vi "Read_Write_Beam_Data.vi"(1 "Beam Data In":T2={"Vg1 (Green 1 dir. vect.)"=[0.059117350659853476, -0.996541267827751, 0.05840068807144843], "Vg2  (Green 2 dir. vect.)"=[-0.05232536310393669, -0.9971561380468801, -0.054237373935992664], "Vb1 (Blue 1 dir. vect.)"=[-0.052923229613528855, -0.9969242065933935, 0.057803616456121795], "Vb2 (Blue 1 dir. vect.)"=[0.05971521716944564, -0.9967731992812374, -0.05364030232066602], "Porb (Orb XYZ posn. forced coplanar)"=[2201.0738225655555, -1199.3737231995547, 269.758310600838], "Porb (Orb XYZ posn. - allow skew)"=[2200.796256301178, -1199.3740953152687, 270.0329332816893], "Orb posn. uncertainty, +/- dx, dy, dz"=[0.13878313218879157, 0.00018605785703584843, 0.13731134042564008], "Vp (Actual Probe dir. vect)"=[0.003406702197773746, -0.9999920168246164, 0.0020882210543692924], "Yaw (deg)"=89.80480953887573, "Pitch (deg)"=0.11964634006213794, "In-Plane Roll (deg)"=45.305328966424156, "Beam Half Angle (deg)"=4.544091484248422, "B1 Close P11"=[0.0, 0.0, 0.0], "B1 Far P12"=[2158.01, -491.04, 229.28], "B2 Close P22"=[2158.01, -491.04, 229.28], "B2 Far P21"=[2158.01, -491.04, 229.28], "Projected Roll (deg)"=0.0, "Green Velocity Vector"=[0.0, 0.0, 0.0], "Blue Velocity Vector"=[0.0, 0.0, 0.0], "Probe is facing...."="-", "Calculation Method"=""} {"Vp (Actual Probe dir. vect)" format="%#_6f"; "Vg2  (Green 2 dir. vect.)" format="%#_6f"; "Vg1 (Green 1 dir. vect.)" format="%#_6f"}, 2 "Mode":T1(ring)) -> (0 "Beam Data Out":T2={"Vg1 (Green 1 dir. vect.)"=[0.059117350659853476, -0.996541267827751, 0.05840068807144843], "Vg2  (Green 2 dir. vect.)"=[-0.05232536310393669, -0.9971561380468801, -0.054237373935992664], "Vb1 (Blue 1 dir. vect.)"=[-0.052923229613528855, -0.9969242065933935, 0.057803616456121795], "Vb2 (Blue 1 dir. vect.)"=[0.05971521716944564, -0.9967731992812374, -0.05364030232066602], "Porb (Orb XYZ posn. forced coplanar)"=[2201.0738225655555, -1199.3737231995547, 269.758310600838], "Porb (Orb XYZ posn. - allow skew)"=[2200.796256301178, -1199.3740953152687, 270.0329332816893], "Orb posn. uncertainty, +/- dx, dy, dz"=[0.13878313218879157, 0.00018605785703584843, 0.13731134042564008], "Vp (Actual Probe dir. vect)"=[0.003406702197773746, -0.9999920168246164, 0.0020882210543692924], "Yaw (deg)"=89.80480953887573, "Pitch (deg)"=0.11964634006213794, "In-Plane Roll (deg)"=45.305328966424156, "Beam Half Angle (deg)"=4.544091484248422, "B1 Close P11"=[0.0, 0.0, 0.0], "B1 Far P12"=[2158.01, -491.04, 229.28], "B2 Close P22"=[2158.01, -491.04, 229.28], "B2 Far P21"=[2158.01, -491.04, 229.28], "Projected Roll (deg)"=0.0, "Green Velocity Vector"=[0.0, 0.0, 0.0], "Blue Velocity Vector"=[0.0, 0.0, 0.0], "Probe is facing...."="-", "Calculation Method"=""} {"Vp (Actual Probe dir. vect)" format="%#_6f"; "Vg2  (Green 2 dir. vect.)" format="%#_6f"; "Vg1 (Green 1 dir. vect.)" format="%#_6f"})   [LabVIEW 2010]
uses:
  Controls/LDA_Beam_Cluster.ctl
  File/Setup_Filetype.ctl
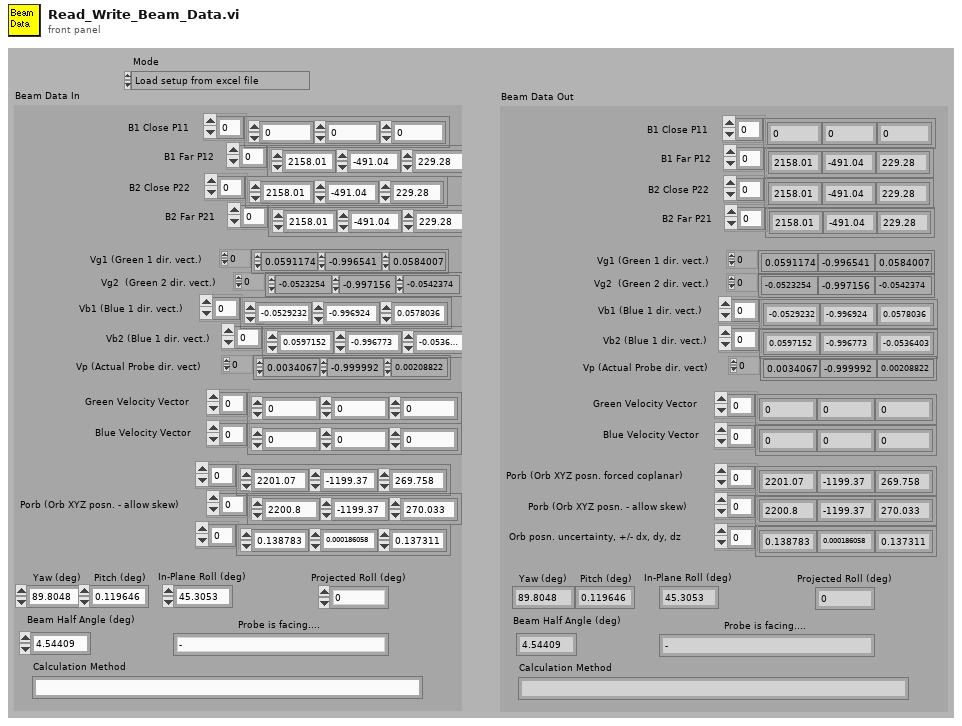
[diagram p1: front panel]
types:
  T1 = enum16{"Load setup from excel file", "Save setup to excel file"}
  T2 = typedef "LDA_Beam_Cluster.ctl" = cluster{"Vg1 (Green 1 dir. vect.)":dbl[], "Vg2  (Green 2 dir. vect.)":dbl[], "Vb1 (Blue 1 dir. vect.)":dbl[], "Vb2 (Blue 1 dir. vect.)":dbl[], "Porb (Orb XYZ posn. forced coplanar)":dbl[], "Porb (Orb XYZ posn. - allow skew)":dbl[], "Orb posn. uncertainty, +/- dx, dy, dz":dbl[], "Vp (Actual Probe dir. vect)":dbl[], "Yaw (deg)":dbl, "Pitch (deg)":dbl, "In-Plane Roll (deg)":dbl, "Beam Half Angle (deg)":dbl, "B1 Close P11":dbl[], "B1 Far P12":dbl[], "B2 Close P22":dbl[], "B2 Far P21":dbl[], "Projected Roll (deg)":dbl, "Green Velocity Vector":dbl[], "Blue Velocity Vector":dbl[], "Probe is facing....":string, "Calculation Method":string}
  T3 = typedef "Setup_Filetype.ctl" = enum16{"Measurement Setups", "Calibration Setups", "General", "Results File Plotter Setups", "Speed Calib Tweaks"}
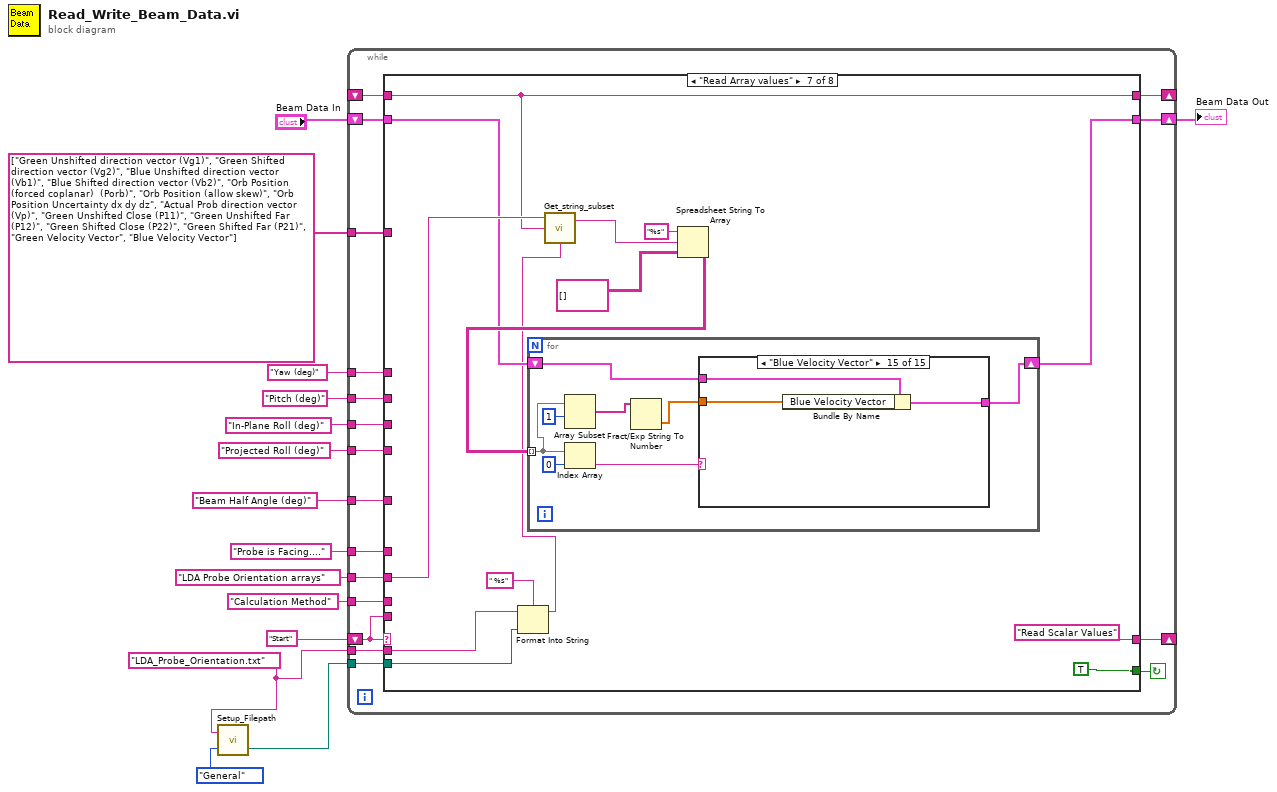
[diagram p0: block diagram]
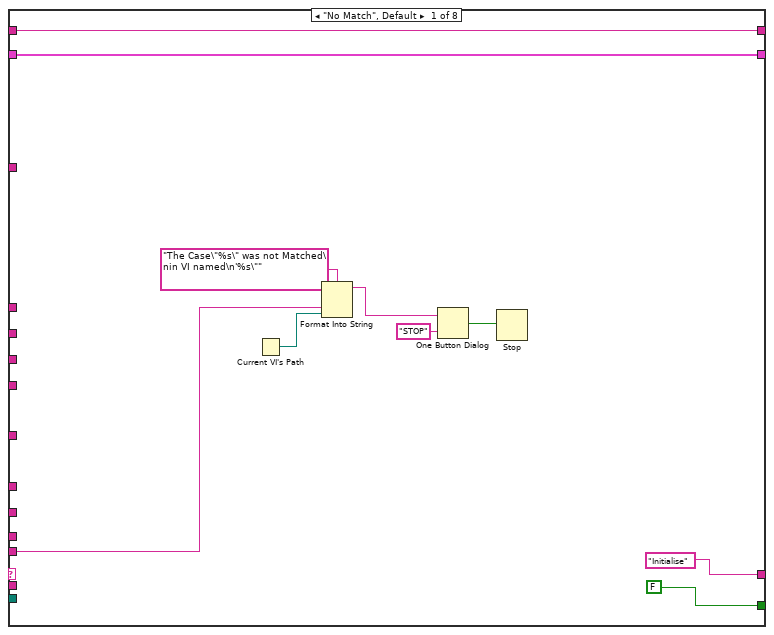
[diagram p2: hidden frame]
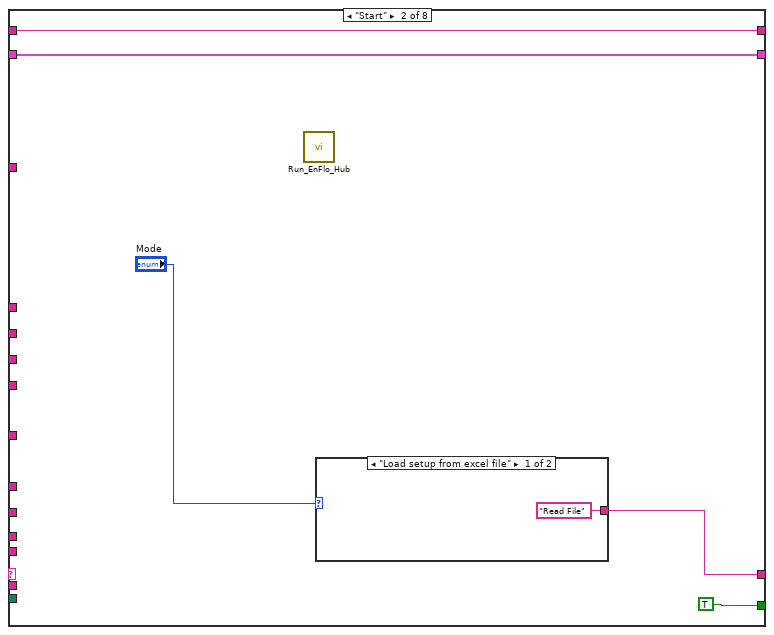
[diagram p3: hidden frame]
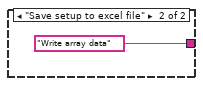
[diagram p4: hidden frame]
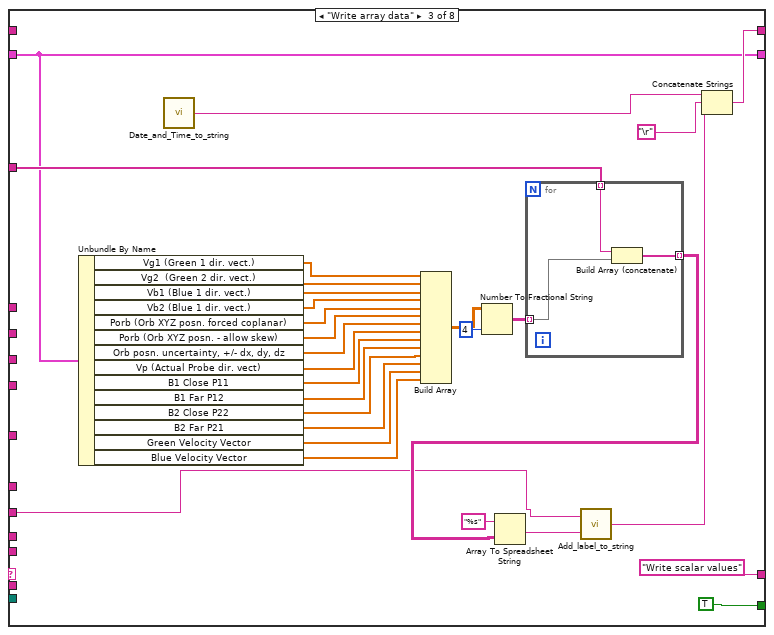
[diagram p5: hidden frame]
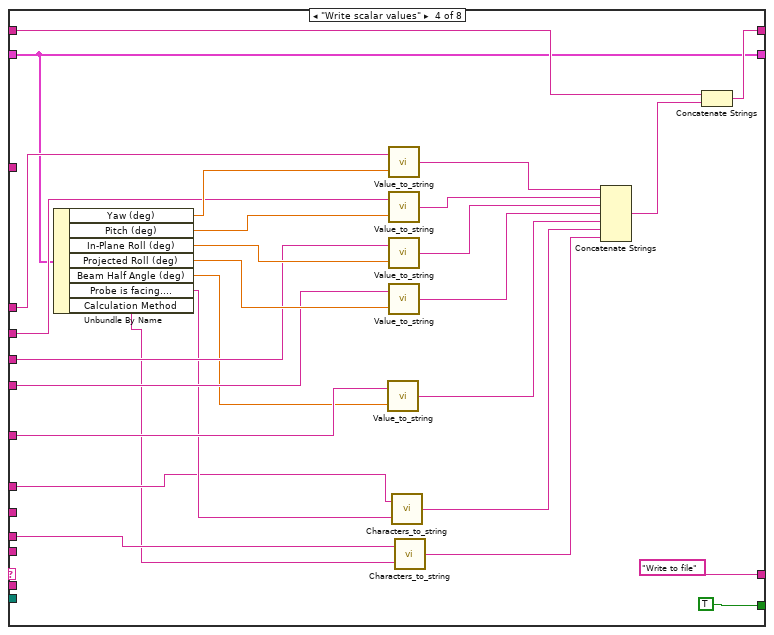
[diagram p6: hidden frame]
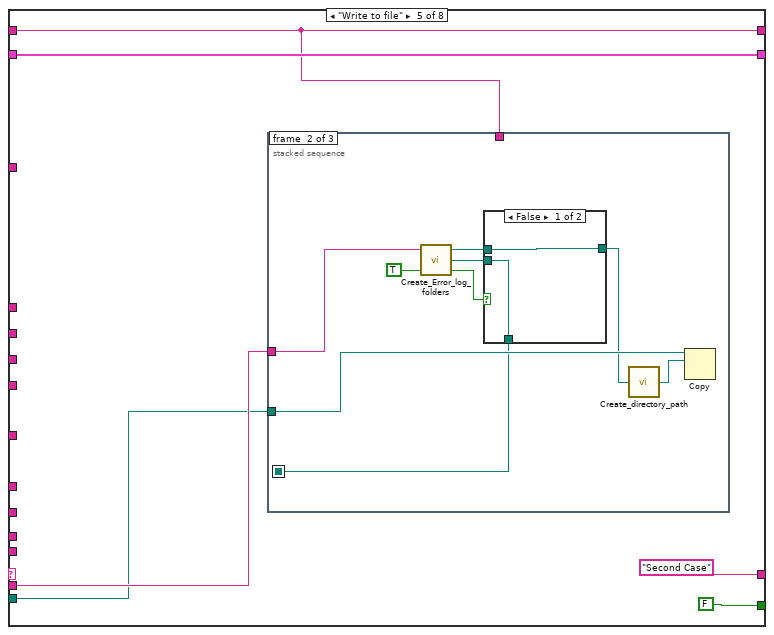
[diagram p7: hidden frame]
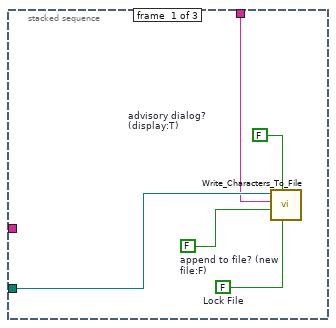
[diagram p8: hidden frame]
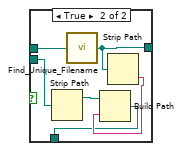
[diagram p9: hidden frame]
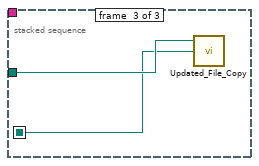
[diagram p10: hidden frame]
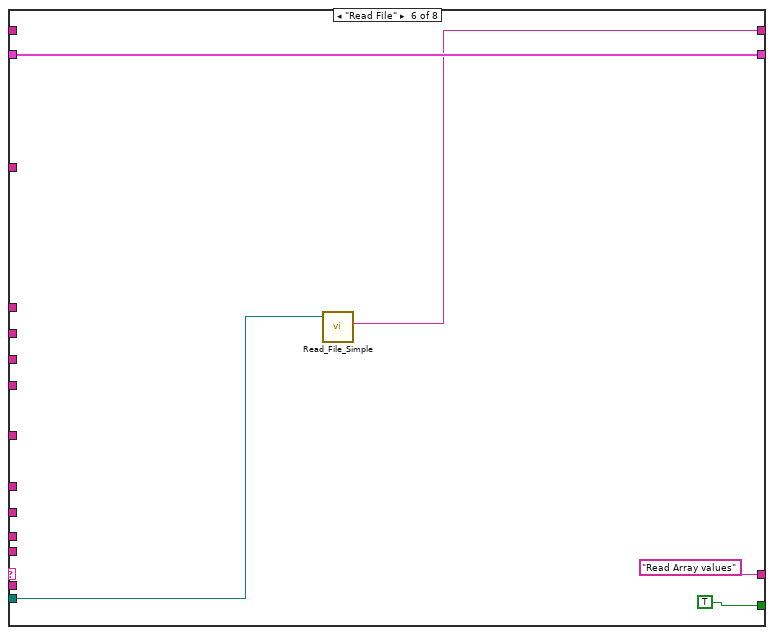
[diagram p11: hidden frame]
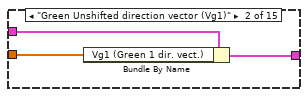
[diagram p13: hidden frame]
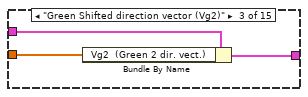
[diagram p14: hidden frame]
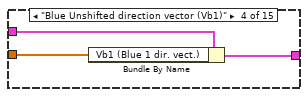
[diagram p15: hidden frame]
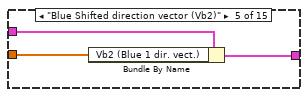
[diagram p16: hidden frame]
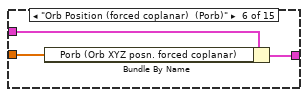
[diagram p17: hidden frame]
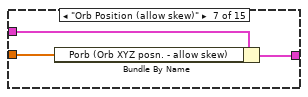
[diagram p18: hidden frame]
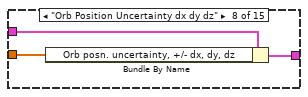
[diagram p19: hidden frame]
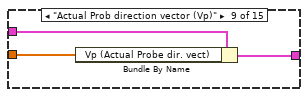
[diagram p20: hidden frame]
diagram:
  w2 = "LDA_Probe_Orientation.txt" ("name or relative path")
  n1 = call "Setup_Filepath.vi"("Setup File Type"=Setup_Filetype."General", "Filename in"=w2) -> ("Filename Out"=w1:path)  [unwired: 1 out]
  n2 = while {
    shift-left: "Start" -> [w31]
    shift-right: [w32] -> _
    shift-right: [w26] -> w13
    shift-left: "Beam Data In" -> [w30]
    shift-right: [w28] -> _
    shift-left: _ -> [w27]
    tunnel: string[] ["Green Unshifted direction vector (Vg1)", "Green Shifted direction vector (Vg2)", "Blue Unshifted direction vector (Vb1)", "Blue Shifted direction vector (Vb2)", "Orb Position (forced coplanar)  (Porb)", "Orb Position (allow skew)", "Orb Position Uncertainty dx dy dz", "Actual Prob direction vector (Vp)", "Green Unshifted Close (P11)", "Green Unshifted Far (P12)", "Green Shifted Close (P22)", "Green Shifted Far (P21)", "Green Velocity Vector", "Blue Velocity Vector"] -> [w29]
    tunnel: "Yaw (deg)" -> [w25]
    tunnel: "Pitch (deg)" -> [w24]
    tunnel: "In-Plane Roll (deg)" -> [w23]
    tunnel: "Projected Roll (deg)" -> [w22]
    tunnel: "LDA Probe Orientation arrays" ("File Label") -> [w21]
    tunnel: "Beam Half Angle (deg)" -> [w20]
    tunnel: "Probe is Facing...." -> [w19]
    tunnel: "Calculation Method" -> [w18]
    tunnel: w1 -> [w17]
    tunnel: w2 -> [w16]
    stop <- w33 continue-if-true
    n3 = case shown="\"Read Array values\"" w31 {
      tunnel: [FALSE TRUE TRUE TRUE FALSE TRUE TRUE FALSE] -> w33
      tunnel: ["Initialise" w44 "Write scalar values" "Write to file" "Second Case" "Read Array values" "Read Scalar Values" "End"] -> w32
      tunnel: w31 -> [w38 _ _ _ _ _ _ _]
      tunnel: w30 -> [w34 w46 w59 w92 w113 w142 w151 w225]
      tunnel: w29 -> [_ _ w66 _ _ _ _ _]
      tunnel: [w35 w47 w61 w107 w112 w141 w149 w212] -> w28
      tunnel: w27 -> [w35 w47 _ w102 w112 _ w149 w212]
      tunnel: [w34 w46 w59 w92 w113 w142 w150 w217] -> w26
      tunnel: w25 -> [_ _ _ w96 _ _ _ w226]
      tunnel: w24 -> [_ _ _ w95 _ _ _ w224]
      tunnel: w23 -> [_ _ _ w94 _ _ _ w223]
      tunnel: w22 -> [_ _ _ w93 _ _ _ w222]
      tunnel: w21 -> [_ _ w60 _ _ _ w156 _]
      tunnel: w20 -> [_ _ _ w91 _ _ _ w216]
      tunnel: w19 -> [_ _ _ w87 _ _ _ w214]
      tunnel: w18 -> [_ _ _ w85 _ _ _ w211]
      tunnel: w17 -> [_ _ _ _ w110 w140 w148 _]
      tunnel: w16 -> [_ _ _ _ w111 _ w146 _]
      frame "No Match", Default {
        n4 = Current VI's Path() -> (path=w37:path)
        n5 = Format Into String(format string="The Case\"%s\" was not Matched\nin VI named\n'%s\"" ("Format String"), w38, w37) -> (resulting string=w41:string)  [unwired: 2 in, 1 out]
        n6 = One Button Dialog(message=w41, button name ("OK")="STOP") -> (true=w39:bool)
        n7 = Stop(stop? (T)=w39) -> ()
      }
      frame "Start" {
        n8 = call "Run_EnFlo_Hub.vi"() -> ()  [unwired: 8 out]
        n9 = case shown="\"Load setup from excel file\"" "Mode" {
          tunnel: ["Read File" "Write array data"] -> w44
          frame "Load setup from excel file" {
          }
          frame "Save setup to excel file" {
          }
        }
      }
      frame "Write array data" {
        n10 = Unbundle By Name(w59) -> ("Vg1 (Green 1 dir. vect.)"=w67:dbl[], "Vg2  (Green 2 dir. vect.)"=w68:dbl[], "Vb1 (Blue 1 dir. vect.)"=w69:dbl[], "Vb2 (Blue 1 dir. vect.)"=w70:dbl[], "Porb (Orb XYZ posn. forced coplanar)"=w71:dbl[], "Porb (Orb XYZ posn. - allow skew)"=w72:dbl[], "Orb posn. uncertainty, +/- dx, dy, dz"=w73:dbl[], "Vp (Actual Probe dir. vect)"=w74:dbl[], "B1 Close P11"=w56:dbl[], "B1 Far P12"=w55:dbl[], "B2 Close P22"=w54:dbl[], "B2 Far P21"=w53:dbl[], "Green Velocity Vector"=w52:dbl[], "Blue Velocity Vector"=w51:dbl[])
        n11 = call "Date_and_Time_to_string.vi"() -> ("Date and time (spreadsheet)"=w62:string)
        n12 = Build Array(w67, w68, w69, w70, w71, w72, w73, w74, w56, w55, w54, w53, w52, w51) -> (w75:dbl[][])
        n13 = Number To Fractional String(number=w75, precision (6)=i16 4) -> (F-format string=w77:string[][])  [unwired: 2 out]
        n14 = for {
          tunnel: w66 -> [w82] mode=indexing
          tunnel: w77 -> [w81] mode=indexing
          tunnel: [w80] -> w63 mode=indexing
          n15 = Build Array (concatenate)(w82, w81) -> (w80:string[])
        }
        n16 = Array To Spreadsheet String(array=w63, 3:"%s" ("format string")) -> (spreadsheet string=w65:string)  [unwired: 1 out]
        n17 = call "Add_label_to_string.vi"("String to write"=w65, "File Label"=w60) -> ("Output string"=w57:string)
        n18 = Concatenate Strings(w62, "\r", w57) -> (w61:string)
      }
      frame "Write scalar values" {
        n19 = Unbundle By Name(w92) -> ("Yaw (deg)"=w106:dbl, "Pitch (deg)"=w105:dbl, "In-Plane Roll (deg)"=w104:dbl, "Projected Roll (deg)"=w103:dbl, "Beam Half Angle (deg)"=w89:dbl, "Probe is facing...."=w88:string, "Calculation Method"=w84:string)
        n20 = call "Value_to_string.vi"("Value"=w89, "Label for value"=w91) -> ("Output string"=w90:string)  [unwired: 1 in]
        n21 = call "Value_to_string.vi"("Value"=w106, "Label for value"=w96) -> ("Output string"=w101:string)  [unwired: 1 in]
        n22 = call "Value_to_string.vi"("Value"=w105, "Label for value"=w95) -> ("Output string"=w100:string)  [unwired: 1 in]
        n23 = call "Value_to_string.vi"("Value"=w104, "Label for value"=w94) -> ("Output string"=w99:string)  [unwired: 1 in]
        n24 = call "Value_to_string.vi"("Value"=w103, "Label for value"=w93) -> ("Output string"=w98:string)  [unwired: 1 in]
        n25 = call "Characters_to_string.vi"("Characters to write"=w88, "Label for characters"=w87) -> ("Output string"=w86:string)
        n26 = call "Characters_to_string.vi"("Characters to write"=w84, "Label for characters"=w85) -> ("Output string"=w83:string)
        n27 = Concatenate Strings(w101, w100, w99, w98, w90, w86, w83) -> (w97:string)
        n28 = Concatenate Strings(w102, w97) -> (w107:string)
      }
      frame "Write to file" {
        n29 = stacked-sequence {
          seq-local: [_ w123 _] -> [_ _ w138]
          tunnel: w110 -> [w120 w127 w139]
          tunnel: w112 -> [w119 _ _]
          tunnel: w111 -> [_ w128 _]
          frame #0 {
            w116 = FALSE  # advisory dialog? (display:T)
            w117 = FALSE  # append to file? (new file:F)
            w118 = FALSE  # Lock File
            n30 = call "Write_Characters_To_File.vi"("file path (dialog if empty)"=w120, "advisory dialog? (display:T)"=w116, "character string"=w119, "append to file? (new file:F)"=w117, "Lock File"=w118) -> ()  [unwired: 4 out]
          }
          frame #1 {
            n31 = call "Create_Error_log_folders.vi"("Per Day Log File?"=TRUE, "Log Filename"=w128) -> ("exists?"=w129:bool, "Server copy Location"=w124:path, "Local Log File"=w125:path)  [unwired: 1 in]
            n32 = case shown="False" w129 {
              tunnel: [w131 w134] -> w122
              tunnel: w125 -> [w131 w137]
              tunnel: [w130 w132] -> w123
              tunnel: w124 -> [w130 w136]
              frame False {
              }
              frame True {
                n33 = Strip Path(path=w136) -> (stripped path=w135:path)  [unwired: 1 out]
                n34 = call "Find_Unique_Filename.vi"("Path In"=w137) -> ("Unique Path Out"=w134:path)  [unwired: 1 in, 1 out]
                n35 = Strip Path(path=w134) -> (name=w133:string)  [unwired: 1 out]
                n36 = Build Path(base path=w135, name or relative path=w133) -> (appended path=w132:path)
              }
            }
            n37 = call "Create_directory_path.vi"("Path name"=w122) -> ("Path name Out"=w121:path)
            n38 = Copy(10:w121, 11:w127) -> ()  [unwired: 1 in, 5 out]
          }
          frame #2 {
            n39 = call "Updated_File_Copy.vi"("Target Path"=w138, "Source Path"=w139) -> ()  [unwired: 2 out]
          }
        }
      }
      frame "Read File" {
        n40 = call "Read_File_Simple.vi"("Filename"=w140) -> ("string"=w141:string)  [unwired: 2 in, 7 out]
      }
      frame "Read Array values" {
        n41 = Format Into String(format string=" %s", initial string=w146, w148) -> (resulting string=w145:string)  [unwired: 1 in, 1 out]
        n42 = call "Get_string_subset.vi"("String Name"=w145, "String to split"=w149, "File Label"=w156) -> ("Output string"=w155:string)  [unwired: 1 in, 1 out]
        n43 = Spreadsheet String To Array(format string="%s", spreadsheet string=w155, array type (2D Dbl)=string[][] []) -> (array=w152:string[][])  [unwired: 1 out]
        n44 = for {
          shift-right: [w165] -> w150
          shift-left: w151 -> [w166]
          tunnel: w152 -> [w161] mode=indexing
          n45 = Array Subset(array=w161, index=1) -> (w160:string[])  [unwired: 1 in]
          n46 = Index Array(array=w161, index=0) -> (element=w163:string)
          n47 = Fract/Exp String To Number(string=w160) -> (number=w159:dbl[])  [unwired: 4 out]
          n48 = case shown="\"Blue Velocity Vector\"" w163 {
            tunnel: w166 -> [w167 w170 w173 w176 w179 w182 w185 w188 w191 w194 w197 w200 w203 w206 w209]
            tunnel: [w167 w169 w172 w175 w178 w181 w184 w187 w190 w193 w196 w199 w202 w205 w208] -> w165
            tunnel: w159 -> [_ w168 w171 w174 w177 w180 w183 w186 w189 w192 w195 w198 w201 w204 w207]
            frame "False", Default {
            }
            frame "Green Unshifted direction vector (Vg1)" {
              n49 = Bundle By Name(cluster=w170, "Vg1 (Green 1 dir. vect.)"=w168) -> (w169:T2)
            }
            frame "Green Shifted direction vector (Vg2)" {
              n50 = Bundle By Name(cluster=w173, "Vg2  (Green 2 dir. vect.)"=w171) -> (w172:T2)
            }
            frame "Blue Unshifted direction vector (Vb1)" {
              n51 = Bundle By Name(cluster=w176, "Vb1 (Blue 1 dir. vect.)"=w174) -> (w175:T2)
            }
            frame "Blue Shifted direction vector (Vb2)" {
              n52 = Bundle By Name(cluster=w179, "Vb2 (Blue 1 dir. vect.)"=w177) -> (w178:T2)
            }
            frame "Orb Position (forced coplanar)  (Porb)" {
              n53 = Bundle By Name(cluster=w182, "Porb (Orb XYZ posn. forced coplanar)"=w180) -> (w181:T2)
            }
            frame "Orb Position (allow skew)" {
              n54 = Bundle By Name(cluster=w185, "Porb (Orb XYZ posn. - allow skew)"=w183) -> (w184:T2)
            }
            frame "Orb Position Uncertainty dx dy dz" {
              n55 = Bundle By Name(cluster=w188, "Orb posn. uncertainty, +/- dx, dy, dz"=w186) -> (w187:T2)
            }
            frame "Actual Prob direction vector (Vp)" {
              n56 = Bundle By Name(cluster=w191, "Vp (Actual Probe dir. vect)"=w189) -> (w190:T2)
            }
            frame "Green Unshifted Close (P11)" {
              n57 = Bundle By Name(cluster=w194, "B1 Close P11"=w192) -> (w193:T2)
            }
            frame "Green Unshifted Far (P12)" {
              n58 = Bundle By Name(cluster=w197, "B1 Far P12"=w195) -> (w196:T2)
            }
            frame "Green Shifted Close (P22)" {
              n59 = Bundle By Name(cluster=w200, "B2 Close P22"=w198) -> (w199:T2)
            }
            frame "Green Shifted Far (P21)" {
              n60 = Bundle By Name(cluster=w203, "B2 Far P21"=w201) -> (w202:T2)
            }
            frame "Green Velocity Vector" {
              n61 = Bundle By Name(cluster=w206, "Green Velocity Vector"=w204) -> (w205:T2)
            }
            frame "Blue Velocity Vector" {
              n62 = Bundle By Name(cluster=w209, "Blue Velocity Vector"=w207) -> (w208:T2)
            }
          }
        }
      }
      frame "Read Scalar Values" {
        n63 = call "Get_value_from_string.vi"("Input string"=w212, "Variable name"=w226) -> ("Value"=w221:dbl)  [unwired: 1 in, 1 out]
        n64 = call "Get_value_from_string.vi"("Input string"=w212, "Variable name"=w222) -> ("Value"=w220:dbl)  [unwired: 1 in, 1 out]
        n65 = call "Get_value_from_string.vi"("Input string"=w212, "Variable name"=w224) -> ("Value"=w218:dbl)  [unwired: 1 in, 1 out]
        n66 = call "Get_value_from_string.vi"("Input string"=w212, "Variable name"=w223) -> ("Value"=w219:dbl)  [unwired: 1 in, 1 out]
        n67 = call "Get_value_from_string.vi"("Input string"=w212, "Variable name"=w216) -> ("Value"=w215:dbl)  [unwired: 1 in, 1 out]
        n68 = call "Get_Characters_from_string.vi"("Input string"=w212, "Variable name"=w214) -> ("Value"=w213:string)  [unwired: 1 in, 1 out]
        n69 = call "Get_Characters_from_string.vi"("Input string"=w212, "Variable name"=w211) -> ("Value"=w210:string)  [unwired: 1 in, 1 out]
        n70 = Bundle By Name(cluster=w225, "Yaw (deg)"=w221, "Pitch (deg)"=w218, "In-Plane Roll (deg)"=w219, "Projected Roll (deg)"=w220, "Beam Half Angle (deg)"=w215, "Probe is facing...."=w213, "Calculation Method"=w210) -> (w217:T2)
      }
    }
  }
  "Beam Data Out" <- w13
